vi "OP600ZP_DCIR.vi"(3 "tableau":string[][](array[string]), 9 "DCIR_MESURES":T1) -> (2 "Tableau 2":string[][](array[string]), 4 "PASS/FAIL":bool[](array[boolean]))   [LabVIEW 2020]
uses:
  OP600ZP_VGConf.vi
  VG/DCIR@1C.vi
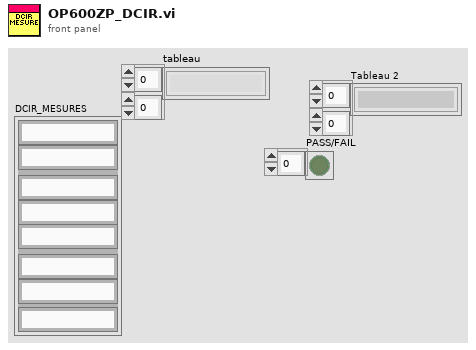
[diagram p1: front panel]
types:
  T1 = cluster{string, string, string, string, string, string, string, string}
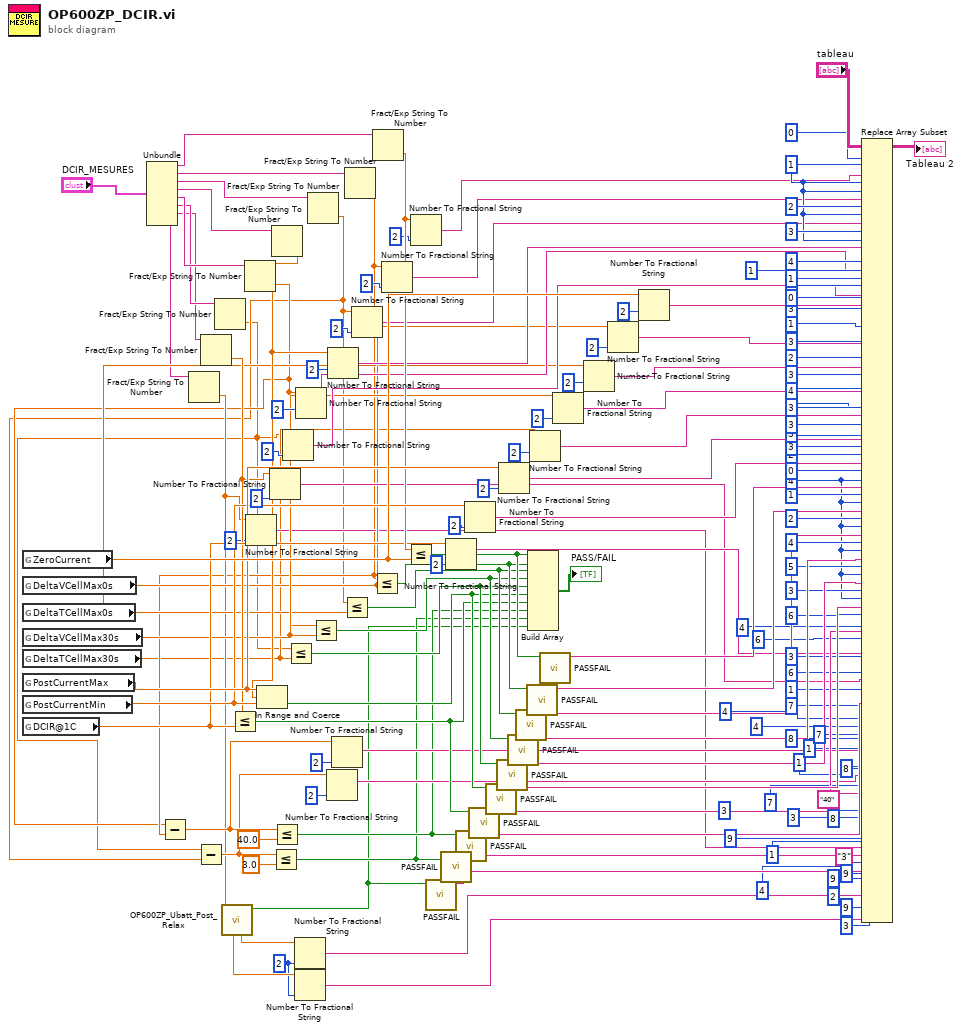
[diagram p0: block diagram]
diagram:
  w12 = i16 2 ("précision (6)")
  w85 = 4 ("indice désactivé (col)")
  w106 = 1 ("indice désactivé (col)")
  n1 = global read "OP600ZP_VGConf.vi" "ZeroCurrent"() -> (w135:dbl)
  n2 = global read "OP600ZP_VGConf.vi" "DeltaVCellMax0s"() -> (w52:dbl)
  n3 = global read "OP600ZP_VGConf.vi" "DeltaTCellMax0s"() -> (w51:dbl)
  n4 = global read "OP600ZP_VGConf.vi" "DeltaVCellMax30s"() -> (w53:dbl)
  n5 = global read "OP600ZP_VGConf.vi" "DeltaTCellMax30s"() -> (w2:dbl)
  n6 = global read "OP600ZP_VGConf.vi" "PostCurrentMax"() -> (w134:dbl)
  n7 = global read "OP600ZP_VGConf.vi" "PostCurrentMin"() -> (w133:dbl)
  n8 = global read "DCIR@1C.vi" "DCIR@1C"() -> (w64:dbl)
  n9 = Unbundle("DCIR_MESURES") -> (w145:string, w144:string, w143:string, w141:string, w73:string, w71:string, w69:string, w24:string)
  n10 = Fract/Exp String To Number(string=w24) -> (number=w22:dbl)  [unwired: 3 in, 1 out]
  n11 = Fract/Exp String To Number(string=w69) -> (number=w59:dbl)  [unwired: 3 in, 1 out]
  n12 = Fract/Exp String To Number(string=w71) -> (number=w1:dbl)  [unwired: 3 in, 1 out]
  n13 = call "OP600ZP_Ubatt_Post_Relax.vi"("Ubatt Post Relax"=w22) -> ("Dans la gamme ?"=w21:bool, "MIN"=w13:dbl, "MAX"=w14:dbl)  [unwired: 7 in, 1 out]
  n14 = Less Or Equal?(x=w59, y=w64) -> (x <= y?=w68:bool)
  n15 = Fract/Exp String To Number(string=w73) -> (number=w4:dbl)  [unwired: 3 in, 1 out]
  n16 = Number To Fractional String(number=w22, precision (6)=i16 2 ("précision (6)")) -> (F-format string=w18:string)  [unwired: 2 in]
  n17 = Number To Fractional String(number=w59, precision (6)=i16 2 ("précision (6)")) -> (F-format string=w56:string)  [unwired: 2 in]
  n18 = Fract/Exp String To Number(string=w141) -> (number=w76:dbl)  [unwired: 3 in, 1 out]
  n19 = In Range and Coerce(upper limit=w134, x=w76, lower limit=w133) -> (In Range?=w98:bool)  [unwired: 1 out]
  n20 = Number To Fractional String(number=w1, precision (6)=i16 2 ("précision (6)")) -> (F-format string=w70:string)  [unwired: 2 in]
  n21 = Less Or Equal?(x=w1, y=w2) -> (x <= y?=w99:bool)
  n22 = Number To Fractional String(number=w13, precision (6)=w12) -> (F-format string=w11:string)  [unwired: 2 in]
  n23 = Number To Fractional String(number=w14, precision (6)=w12) -> (F-format string=w10:string)  [unwired: 2 in]
  n24 = Number To Fractional String(number=w4, precision (6)=i16 2 ("précision (6)")) -> (F-format string=w72:string)  [unwired: 2 in]
  n25 = Fract/Exp String To Number(string=w143) -> (number=w3:dbl)  [unwired: 3 in, 1 out]
  n26 = Subtract(x=w1, y=w3) -> (x-y=w40:dbl)
  n27 = Less Or Equal?(x=w40, y=3.0) -> (x <= y?=w25:bool)
  n28 = Less Or Equal?(x=w4, y=w53) -> (x <= y?=w100:bool)
  n29 = Number To Fractional String(number=w40, precision (6)=i16 2 ("précision (6)")) -> (F-format string=w36:string)  [unwired: 2 in]
  n30 = Number To Fractional String(number=w76, precision (6)=i16 2 ("précision (6)")) -> (F-format string=w75:string)  [unwired: 2 in]
  n31 = Less Or Equal?(x=w3, y=w51) -> (x <= y?=w101:bool)
  n32 = Fract/Exp String To Number(string=w144) -> (number=w5:dbl)  [unwired: 3 in, 1 out]
  n33 = Subtract(x=w4, y=w5) -> (x-y=w41:dbl)
  n34 = Less Or Equal?(x=w41, y=40.0) -> (x <= y?=w26:bool)
  n35 = Number To Fractional String(number=w41, precision (6)=i16 2 ("précision (6)")) -> (F-format string=w39:string)  [unwired: 2 in]
  n36 = Number To Fractional String(number=w3, precision (6)=i16 2 ("précision (6)")) -> (F-format string=w79:string)  [unwired: 2 in]
  n37 = Less Or Equal?(x=w5, y=w52) -> (x <= y?=w102:bool)
  n38 = Fract/Exp String To Number(string=w145) -> (number=w84:dbl)  [unwired: 3 in, 1 out]
  n39 = Number To Fractional String(number=w5, precision (6)=i16 2 ("précision (6)")) -> (F-format string=w81:string)  [unwired: 2 in]
  n40 = Less Or Equal?(x=w84, y=w135) -> (x <= y?=w103:bool)
  n41 = Number To Fractional String(number=w84, precision (6)=i16 2 ("précision (6)")) -> (F-format string=w83:string)  [unwired: 2 in]
  n42 = call <vilib>:"PASSFAIL.vi"("E"=w21) -> ("S"=w17:string)  [unwired: 10 in]
  n43 = call <vilib>:"PASSFAIL.vi"("E"=w25) -> ("S"=w48:string)  [unwired: 10 in]
  n44 = Number To Fractional String(number=w64, precision (6)=i16 2 ("précision (6)")) -> (F-format string=w62:string)  [unwired: 2 in]
  n45 = call <vilib>:"PASSFAIL.vi"("E"=w26) -> ("S"=w49:string)  [unwired: 10 in]
  n46 = Number To Fractional String(number=w133, precision (6)=i16 2 ("précision (6)")) -> (F-format string=w120:string)  [unwired: 2 in]
  n47 = call <vilib>:"PASSFAIL.vi"("E"=w68) -> ("S"=w67:string)  [unwired: 10 in]
  n48 = call <vilib>:"PASSFAIL.vi"("E"=w98) -> ("S"=w87:string)  [unwired: 10 in]
  n49 = call <vilib>:"PASSFAIL.vi"("E"=w99) -> ("S"=w89:string)  [unwired: 10 in]
  n50 = Number To Fractional String(number=w134, precision (6)=i16 2 ("précision (6)")) -> (F-format string=w107:string)  [unwired: 2 in]
  n51 = call <vilib>:"PASSFAIL.vi"("E"=w100) -> ("S"=w91:string)  [unwired: 10 in]
  n52 = call <vilib>:"PASSFAIL.vi"("E"=w101) -> ("S"=w93:string)  [unwired: 10 in]
  n53 = call <vilib>:"PASSFAIL.vi"("E"=w102) -> ("S"=w95:string)  [unwired: 10 in]
  n54 = Build Array(w103, w102, w101, w100, w99, w98, w68, w26, w25, w21) -> (→"PASS/FAIL":bool[])
  n55 = Number To Fractional String(number=w2, precision (6)=i16 2 ("précision (6)")) -> (F-format string=w121:string)  [unwired: 2 in]
  n56 = call <vilib>:"PASSFAIL.vi"("E"=w103) -> ("S"=w97:string)  [unwired: 10 in]
  n57 = Number To Fractional String(number=w53, precision (6)=i16 2 ("précision (6)")) -> (F-format string=w122:string)  [unwired: 2 in]
  n58 = Number To Fractional String(number=w51, precision (6)=i16 2 ("précision (6)")) -> (F-format string=w123:string)  [unwired: 2 in]
  n59 = Number To Fractional String(number=w52, precision (6)=i16 2 ("précision (6)")) -> (F-format string=w124:string)  [unwired: 2 in]
  n60 = Number To Fractional String(number=w135, precision (6)=i16 2 ("précision (6)")) -> (F-format string=w125:string)  [unwired: 2 in]
  n61 = Replace Array Subset(array="tableau", new element #1=w83, index (row) #1=0 ("indice (ligne)"), index (col) #1=w106, new element #2=w81, index (row) #2=w106, index (col) #2=w106, new element #3=w79, index (row) #3=2 ("indice (ligne)"), index (col) #3=w106, new element #4=w75, index (row) #4=3 ("indice (ligne)"), index (col) #4=w106, new element #5=w72, index (row) #5=4 ("indice (ligne)"), index (col) #5=1 ("indice désactivé (col)"), new element #6=w70, index (row) #6=5 ("indice (ligne)"), index (col) #6=1 ("indice désactivé (col)"), new element #7=w125, index (row) #7=0 ("indice (ligne)"), index (col) #7=3 ("indice désactivé (col)"), new element #8=w124, index (row) #8=1 ("indice (ligne)"), index (col) #8=3 ("indice désactivé (col)"), new element #9=w123, index (row) #9=2 ("indice (ligne)"), index (col) #9=3 ("indice désactivé (col)"), new element #10=w122, index (row) #10=4 ("indice (ligne)"), index (col) #10=3 ("indice désactivé (col)"), new element #11=w121, index (row) #11=5 ("indice (ligne)"), index (col) #11=3 ("indice désactivé (col)"), new element #12=w107, index (row) #12=3 ("indice (ligne)"), index (col) #12=3 ("indice désactivé (col)"), new element #13=w120, index (row) #13=3 ("indice (ligne)"), index (col) #13=2 ("indice désactivé (col)"), new element #14=w97, index (row) #14=0 ("indice (ligne)"), index (col) #14=w85, new element #15=w95, index (row) #15=1 ("indice (ligne)"), index (col) #15=w85, new element #16=w93, index (row) #16=2 ("indice (ligne)"), index (col) #16=w85, new element #17=w91, index (row) #17=4 ("indice (ligne)"), index (col) #17=w85, new element #18=w89, index (row) #18=5 ("indice (ligne)"), index (col) #18=w85, new element #19=w87, index (row) #19=3 ("indice (ligne)"), index (col) #19=w85, new element #20=w67, index (row) #20=6 ("indice (ligne)"), index (col) #20=4 ("indice désactivé (col)"), new element #21=w62, index (row) #21=6 ("indice (ligne)"), index (col) #21=3 ("indice désactivé (col)"), new element #22=w56, index (row) #22=6 ("indice (ligne)"), index (col) #22=1 ("indice désactivé (col)"), new element #23=w49, index (row) #23=7 ("indice (ligne)"), index (col) #23=4 ("indice désactivé (col)"), new element #24=w48, index (row) #24=8 ("indice (ligne)"), index (col) #24=4 ("indice désactivé (col)"), new element #25=w39, index (row) #25=7 ("indice (ligne)"), index (col) #25=1 ("indice désactivé (col)"), new element #26=w36, index (row) #26=8 ("indice (ligne)"), index (col) #26=1 ("indice désactivé (col)"), new element #27="40" ("nouvel élément/sous-tableau"), index (row) #27=7 ("indice (ligne)"), index (col) #27=3 ("indice désactivé (col)"), new element #28="3" ("nouvel élément/sous-tableau"), index (row) #28=8 ("indice (ligne)"), index (col) #28=3 ("indice désactivé (col)"), new element #29=w18, index (row) #29=9 ("indice (ligne)"), index (col) #29=1 ("indice désactivé (col)"), new element #30=w17, index (row) #30=9 ("indice (ligne)"), index (col) #30=4 ("indice désactivé (col)"), new element #31=w11, index (row) #31=9 ("indice (ligne)"), index (col) #31=2 ("indice désactivé (col)"), new element #32=w10, index (row) #32=9 ("indice (ligne)"), index (col) #32=3 ("indice désactivé (col)")) -> (→"Tableau 2":string[][])
